vi "LV_Arduino.vi"() -> ()   [LabVIEW 2010]
uses:
  <vilib>/Utility/error.llb/DialogType.ctl
  <vilib>/Instr/_visa.llb/VISA Configure Serial Port (Instr).vi
panel:
  out "Current Valve":dbl
  out "Switch Valve":bool
  in  "Number of Bottles in Linearization":dbl=7.0
  in  "Slope Trigger":bool
  out "Boolean":bool
  in  "Manually Switch Valves":bool
  in  "baud rate (9600)":u32=9600
  in  "Stop Program":bool
  in  "Valve to switch":dbl min=0.0 max=16.0 step=1.0
  in  "VISA resource name":refnum<visa-resource-name>="COM10"
  # "Automatic Linearization"
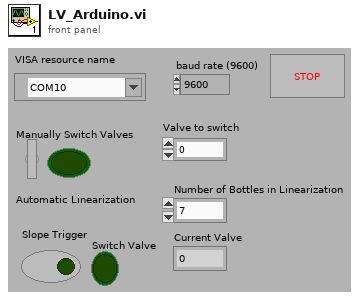
[diagram p1: front panel]
types:
  T1 = typedef "DialogType.ctl" = u16
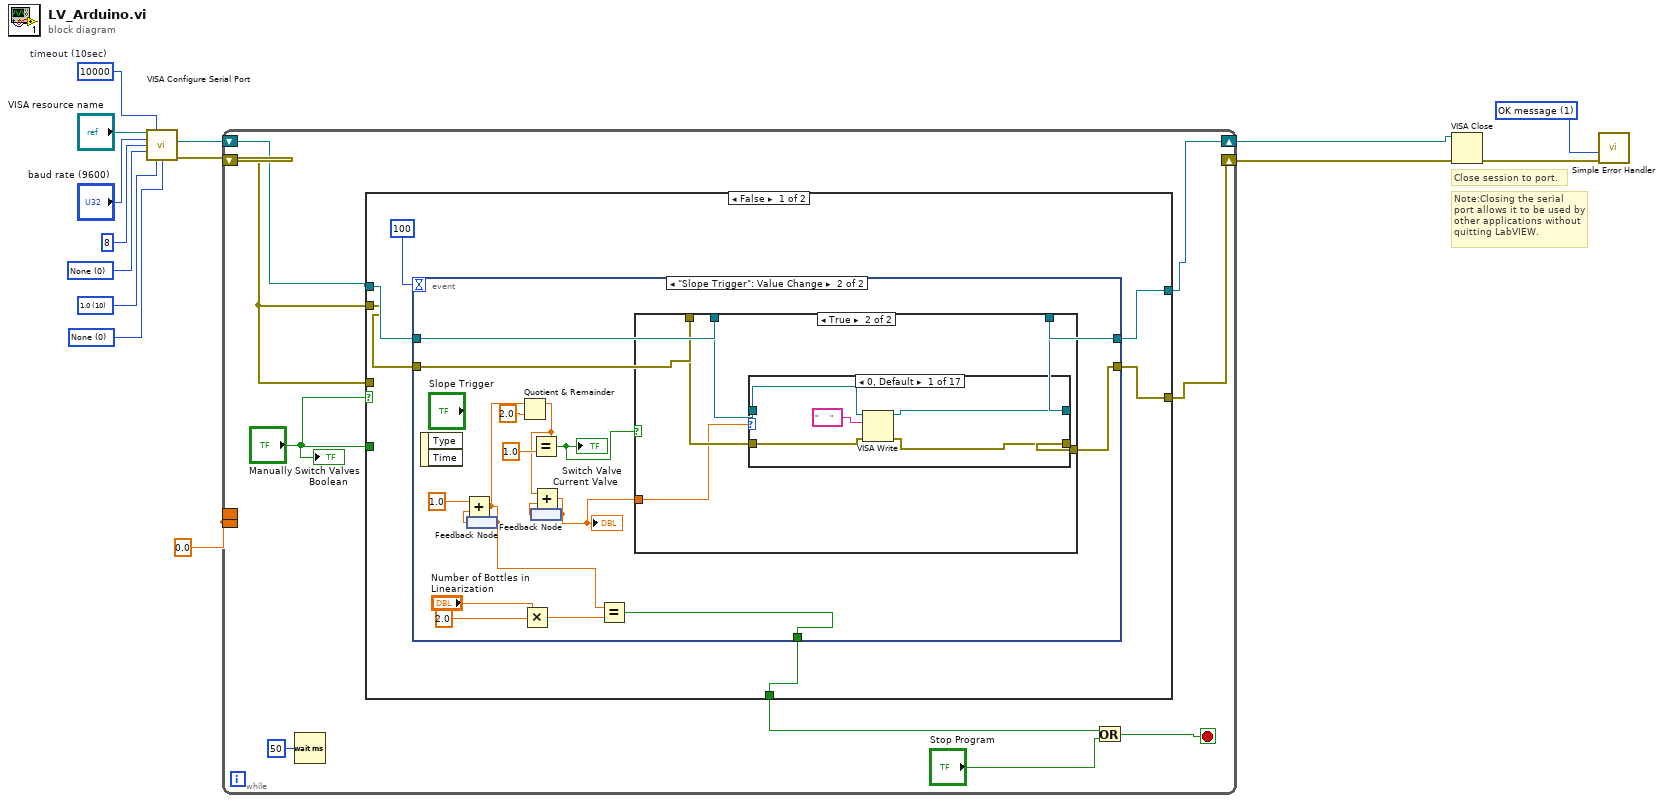
[diagram p0: block diagram]
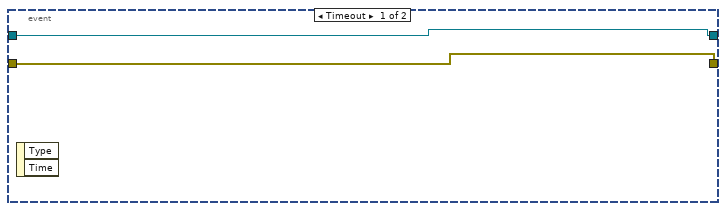
[diagram p2: hidden frame]
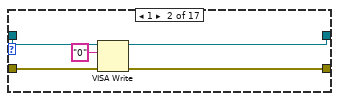
[diagram p4: hidden frame]
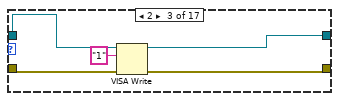
[diagram p5: hidden frame]
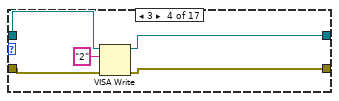
[diagram p6: hidden frame]
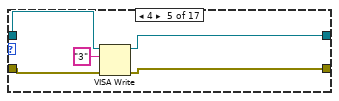
[diagram p7: hidden frame]
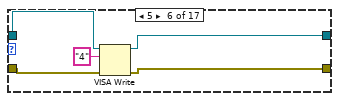
[diagram p8: hidden frame]
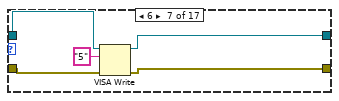
[diagram p9: hidden frame]
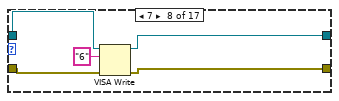
[diagram p10: hidden frame]
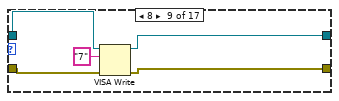
[diagram p11: hidden frame]
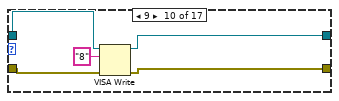
[diagram p12: hidden frame]
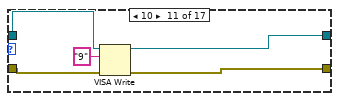
[diagram p13: hidden frame]
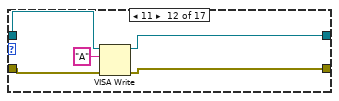
[diagram p14: hidden frame]
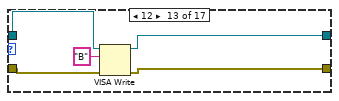
[diagram p15: hidden frame]
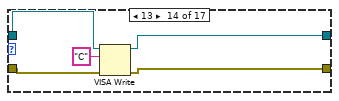
[diagram p16: hidden frame]
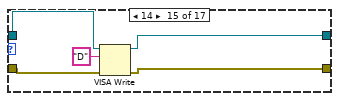
[diagram p17: hidden frame]
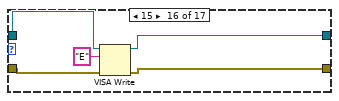
[diagram p18: hidden frame]
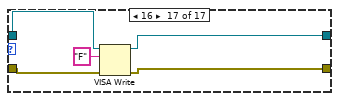
[diagram p19: hidden frame]
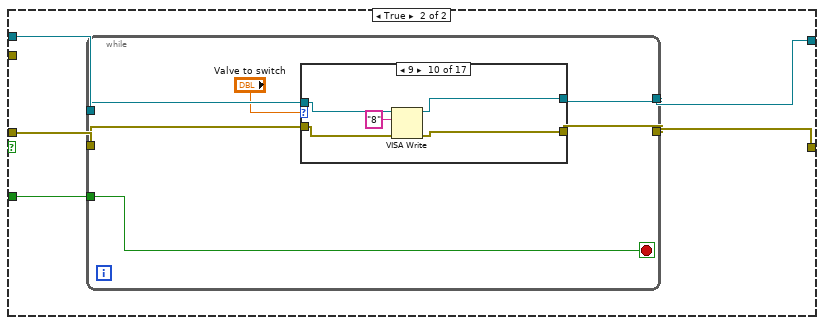
[diagram p20: hidden frame]
diagram:
  w1 = 0.0 ("Value (Signaling)")
  w5 = T1 1 items=["no dialog", "OK message", "continue or stop message", "OK message + warnings", "continue/stop + warnings"] ("type of dialog (OK msg:1)")
  w10 = u16 0 items=["None"=0, "XON/XOFF"=1, "RTS/CTS"=2, "DTR/DSR"=4] ("flow control")
  w11 = u16 10 items=["1.0"=10, "1.5"=15, "2.0"=20] ("stop bits")
  w13 = u16 0 items=["None", "Odd", "Even", "Mark", "Space"] ("parity")
  w12 = u32 10000  # timeout (10sec)
  # "Note:Closing the serial port allows it to be used by other applications without\nquitting LabVIEW."
  # "Close session to port."
  n1 = call-poly "VISA Configure Serial Port"("VISA resource name"="VISA resource name", "timeout (10sec)"=w12, "baud rate (9600)"="baud rate (9600)", "data bits (8)"=u16 8 ("data bits"), "parity (0:none)"=w13, "stop bits (10: 1 bit)"=w11, "flow control (0:none)"=w10) -> ("VISA resource name out"=w4:refnum<visa-resource-name>, "error out"=w2:errorcluster)  [unwired: 2 in, 5 out]
  n2 = while {
    shift-right: [w21] -> w3
    shift-left: w2 -> [w20]
    shift-right: [w22] -> w6
    shift-left: w4 -> [w23]
    border: w1 -> [_]
    border: w1 -> [_]
    stop <- w16 stop-if-true
    n3 = Wait (ms)(milliseconds to wait=u32 50) -> ()  [unwired: 1 out]
    n4 = case shown="False" "Manually Switch Valves" {
      tunnel: w23 -> [w27 w145]
      tunnel: w20 -> [_ w144]
      tunnel: [w26 w142] -> w22
      tunnel: [w25 w141] -> w21
      tunnel: w20 -> [w24 _]
      tunnel: "Manually Switch Valves" -> [_ w143]
      tunnel: [w29 _] -> w18
      frame False {
        n5 = event shown="[1] \"Slope Trigger\": Value Change" {
          selector: _ -> [_ _]
          dyn-events: _ -> [_ _]
          timeout: 100 -> [_ _]
          tunnel: [_ w32] -> w29
          tunnel: [w31 w41] -> w26
          tunnel: w27 -> [w31 w43]
          tunnel: w24 -> [w30 w42]
          tunnel: [w30 w40] -> w25
          event Timeout {
            n6 = event-data() -> ()  [unwired: 1 in, 2 out]
          }
          event "Slope Trigger": Value Change {
            n7 = event-data() -> ()  [unwired: 1 in, 2 out]
            n8 = feedback #1() -> (w48:dbl)
            n9 = Add(x=1.0, y=w48) -> (x+y=w39:dbl)
            n10 = feedback-in #1(w39) -> ()
            n11 = Quotient & Remainder(x=w39, y=2.0) -> (x-y*floor(x/y)=w37:dbl)  [unwired: 1 out]
            n12 = Multiply(x="Number of Bottles in Linearization", y=2.0) -> (x*y=w33:dbl)
            n13 = Equal?(x=w37, y=1.0) -> (x = y?=w44:bool)
            "Switch Valve" <- w44
            n14 = feedback #2() -> (w38:dbl)
            n15 = Add(x=w37, y=w38) -> (x+y=w36:dbl)
            "Current Valve" <- w36
            n16 = feedback-in #2(w36) -> ()
            n17 = Equal?(x=w39, y=w33) -> (x = y?=w32:bool)
            n18 = case shown="True" w44 {
              tunnel: w43 -> [w49 w55]
              tunnel: w42 -> [w50 w54]
              tunnel: [w49 w53] -> w41
              tunnel: [w50 w52] -> w40
              tunnel: w36 -> [_ w51]
              frame False {
              }
              frame True {
                n19 = case shown="0, Default" w51 {
                  tunnel: [w59 w65 w69 w74 w79 w84 w89 w94 w99 w104 w107 w114 w119 w124 w129 w134 w139] -> w53
                  tunnel: [w58 w64 w68 w73 w78 w83 w88 w93 w98 w103 w106 w113 w118 w123 w128 w133 w138] -> w52
                  tunnel: w55 -> [w57 w62 w67 w72 w77 w82 w87 w92 w97 w102 w109 w112 w117 w122 w127 w132 w137]
                  tunnel: w54 -> [w56 w61 w66 w71 w76 w81 w86 w91 w96 w101 w108 w111 w116 w121 w126 w131 w136]
                  frame 0, Default {
                    n20 = VISA Write(VISA resource name=w57, write buffer="      ", error in (no error)=w56) -> (VISA resource name out=w59:refnum<visa-resource-name>, error out=w58:errorcluster)  [unwired: 1 out]
                  }
                  frame 1 {
                    n21 = VISA Write(VISA resource name=w62, write buffer="0", error in (no error)=w61) -> (VISA resource name out=w65:refnum<visa-resource-name>, error out=w64:errorcluster)  [unwired: 1 out]
                  }
                  frame 2 {
                    n22 = VISA Write(VISA resource name=w67, write buffer="1", error in (no error)=w66) -> (VISA resource name out=w69:refnum<visa-resource-name>, error out=w68:errorcluster)  [unwired: 1 out]
                  }
                  frame 3 {
                    n23 = VISA Write(VISA resource name=w72, write buffer="2", error in (no error)=w71) -> (VISA resource name out=w74:refnum<visa-resource-name>, error out=w73:errorcluster)  [unwired: 1 out]
                  }
                  frame 4 {
                    n24 = VISA Write(VISA resource name=w77, write buffer="3", error in (no error)=w76) -> (VISA resource name out=w79:refnum<visa-resource-name>, error out=w78:errorcluster)  [unwired: 1 out]
                  }
                  frame 5 {
                    n25 = VISA Write(VISA resource name=w82, write buffer="4", error in (no error)=w81) -> (VISA resource name out=w84:refnum<visa-resource-name>, error out=w83:errorcluster)  [unwired: 1 out]
                  }
                  frame 6 {
                    n26 = VISA Write(VISA resource name=w87, write buffer="5", error in (no error)=w86) -> (VISA resource name out=w89:refnum<visa-resource-name>, error out=w88:errorcluster)  [unwired: 1 out]
                  }
                  frame 7 {
                    n27 = VISA Write(VISA resource name=w92, write buffer="6", error in (no error)=w91) -> (VISA resource name out=w94:refnum<visa-resource-name>, error out=w93:errorcluster)  [unwired: 1 out]
                  }
                  frame 8 {
                    n28 = VISA Write(VISA resource name=w97, write buffer="7", error in (no error)=w96) -> (VISA resource name out=w99:refnum<visa-resource-name>, error out=w98:errorcluster)  [unwired: 1 out]
                  }
                  frame 9 {
                    n29 = VISA Write(VISA resource name=w102, write buffer="8", error in (no error)=w101) -> (VISA resource name out=w104:refnum<visa-resource-name>, error out=w103:errorcluster)  [unwired: 1 out]
                  }
                  frame 10 {
                    n30 = VISA Write(VISA resource name=w109, write buffer="9", error in (no error)=w108) -> (VISA resource name out=w107:refnum<visa-resource-name>, error out=w106:errorcluster)  [unwired: 1 out]
                  }
                  frame 11 {
                    n31 = VISA Write(VISA resource name=w112, write buffer="A", error in (no error)=w111) -> (VISA resource name out=w114:refnum<visa-resource-name>, error out=w113:errorcluster)  [unwired: 1 out]
                  }
                  frame 12 {
                    n32 = VISA Write(VISA resource name=w117, write buffer="B", error in (no error)=w116) -> (VISA resource name out=w119:refnum<visa-resource-name>, error out=w118:errorcluster)  [unwired: 1 out]
                  }
                  frame 13 {
                    n33 = VISA Write(VISA resource name=w122, write buffer="C", error in (no error)=w121) -> (VISA resource name out=w124:refnum<visa-resource-name>, error out=w123:errorcluster)  [unwired: 1 out]
                  }
                  frame 14 {
                    n34 = VISA Write(VISA resource name=w127, write buffer="D", error in (no error)=w126) -> (VISA resource name out=w129:refnum<visa-resource-name>, error out=w128:errorcluster)  [unwired: 1 out]
                  }
                  frame 15 {
                    n35 = VISA Write(VISA resource name=w132, write buffer="E", error in (no error)=w131) -> (VISA resource name out=w134:refnum<visa-resource-name>, error out=w133:errorcluster)  [unwired: 1 out]
                  }
                  frame 16 {
                    n36 = VISA Write(VISA resource name=w137, write buffer="F", error in (no error)=w136) -> (VISA resource name out=w139:refnum<visa-resource-name>, error out=w138:errorcluster)  [unwired: 1 out]
                  }
                }
              }
            }
          }
        }
      }
      frame True {
        n37 = while {
          tunnel: w145 -> [w150]
          tunnel: w144 -> [w149]
          tunnel: w143 -> [w151]
          tunnel: [w147] -> w142
          tunnel: [w146] -> w141
          stop <- w151 stop-if-true
          n38 = case shown="9" "Valve to switch" {
            tunnel: [w155 w161 w165 w170 w175 w180 w185 w190 w195 w200 w205 w210 w215 w220 w225 w230 w235] -> w147
            tunnel: [w154 w160 w164 w169 w174 w179 w184 w189 w194 w199 w204 w209 w214 w219 w224 w229 w234] -> w146
            tunnel: w150 -> [w153 w158 w163 w168 w173 w178 w183 w188 w193 w198 w203 w208 w213 w218 w223 w228 w233]
            tunnel: w149 -> [w152 w157 w162 w167 w172 w177 w182 w187 w192 w197 w202 w207 w212 w217 w222 w227 w232]
            frame 0, Default {
              n39 = VISA Write(VISA resource name=w153, write buffer="      ", error in (no error)=w152) -> (VISA resource name out=w155:refnum<visa-resource-name>, error out=w154:errorcluster)  [unwired: 1 out]
            }
            frame 1 {
              n40 = VISA Write(VISA resource name=w158, write buffer="0", error in (no error)=w157) -> (VISA resource name out=w161:refnum<visa-resource-name>, error out=w160:errorcluster)  [unwired: 1 out]
            }
            frame 2 {
              n41 = VISA Write(VISA resource name=w163, write buffer="1", error in (no error)=w162) -> (VISA resource name out=w165:refnum<visa-resource-name>, error out=w164:errorcluster)  [unwired: 1 out]
            }
            frame 3 {
              n42 = VISA Write(VISA resource name=w168, write buffer="2", error in (no error)=w167) -> (VISA resource name out=w170:refnum<visa-resource-name>, error out=w169:errorcluster)  [unwired: 1 out]
            }
            frame 4 {
              n43 = VISA Write(VISA resource name=w173, write buffer="3", error in (no error)=w172) -> (VISA resource name out=w175:refnum<visa-resource-name>, error out=w174:errorcluster)  [unwired: 1 out]
            }
            frame 5 {
              n44 = VISA Write(VISA resource name=w178, write buffer="4", error in (no error)=w177) -> (VISA resource name out=w180:refnum<visa-resource-name>, error out=w179:errorcluster)  [unwired: 1 out]
            }
            frame 6 {
              n45 = VISA Write(VISA resource name=w183, write buffer="5", error in (no error)=w182) -> (VISA resource name out=w185:refnum<visa-resource-name>, error out=w184:errorcluster)  [unwired: 1 out]
            }
            frame 7 {
              n46 = VISA Write(VISA resource name=w188, write buffer="6", error in (no error)=w187) -> (VISA resource name out=w190:refnum<visa-resource-name>, error out=w189:errorcluster)  [unwired: 1 out]
            }
            frame 8 {
              n47 = VISA Write(VISA resource name=w193, write buffer="7", error in (no error)=w192) -> (VISA resource name out=w195:refnum<visa-resource-name>, error out=w194:errorcluster)  [unwired: 1 out]
            }
            frame 9 {
              n48 = VISA Write(VISA resource name=w198, write buffer="8", error in (no error)=w197) -> (VISA resource name out=w200:refnum<visa-resource-name>, error out=w199:errorcluster)  [unwired: 1 out]
            }
            frame 10 {
              n49 = VISA Write(VISA resource name=w203, write buffer="9", error in (no error)=w202) -> (VISA resource name out=w205:refnum<visa-resource-name>, error out=w204:errorcluster)  [unwired: 1 out]
            }
            frame 11 {
              n50 = VISA Write(VISA resource name=w208, write buffer="A", error in (no error)=w207) -> (VISA resource name out=w210:refnum<visa-resource-name>, error out=w209:errorcluster)  [unwired: 1 out]
            }
            frame 12 {
              n51 = VISA Write(VISA resource name=w213, write buffer="B", error in (no error)=w212) -> (VISA resource name out=w215:refnum<visa-resource-name>, error out=w214:errorcluster)  [unwired: 1 out]
            }
            frame 13 {
              n52 = VISA Write(VISA resource name=w218, write buffer="C", error in (no error)=w217) -> (VISA resource name out=w220:refnum<visa-resource-name>, error out=w219:errorcluster)  [unwired: 1 out]
            }
            frame 14 {
              n53 = VISA Write(VISA resource name=w223, write buffer="D", error in (no error)=w222) -> (VISA resource name out=w225:refnum<visa-resource-name>, error out=w224:errorcluster)  [unwired: 1 out]
            }
            frame 15 {
              n54 = VISA Write(VISA resource name=w228, write buffer="E", error in (no error)=w227) -> (VISA resource name out=w230:refnum<visa-resource-name>, error out=w229:errorcluster)  [unwired: 1 out]
            }
            frame 16 {
              n55 = VISA Write(VISA resource name=w233, write buffer="F", error in (no error)=w232) -> (VISA resource name out=w235:refnum<visa-resource-name>, error out=w234:errorcluster)  [unwired: 1 out]
            }
          }
        }
      }
    }
    n56 = Or(x=w18, y="Stop Program") -> (x .or. y?=w16:bool)
    "Boolean" <- "Manually Switch Valves"
  }
  n57 = VISA Close(VISA resource name=w6, error in (no error)=w3) -> (error out=w8:errorcluster)
  n58 = call <vilib>:"Simple Error Handler.vi"("type of dialog (OK msg:1)"=w5, "error in (no error)"=w8) -> ()  [unwired: 8 out]
